vi "partsTracking_Create.vi"(6 "error in (no error)":errorcluster, 7 "dim":i32, 8 "index":i32, 9 "reference in":refnum<class "partsTracking.lvclass">) -> (0 "error out":errorcluster, 3 "reference out":refnum<class "partsTracking.lvclass">)   [LabVIEW 2016, in "partsTracking.lvclass"]
doc: "Constructor."
uses:
  partsTracking.lvclass
  C:/Program Files (x86)/National Instruments/LabVIEW 2016/vi.lib/addons/_AddQ/G#Object/G#Object.lvclass
  <vilib>/addons/_AddQ/G#Object/utils/G#Object_CreateMethod.ctl
  <vilib>/addons/_AddQ/G#Object/G#Object.lvclass
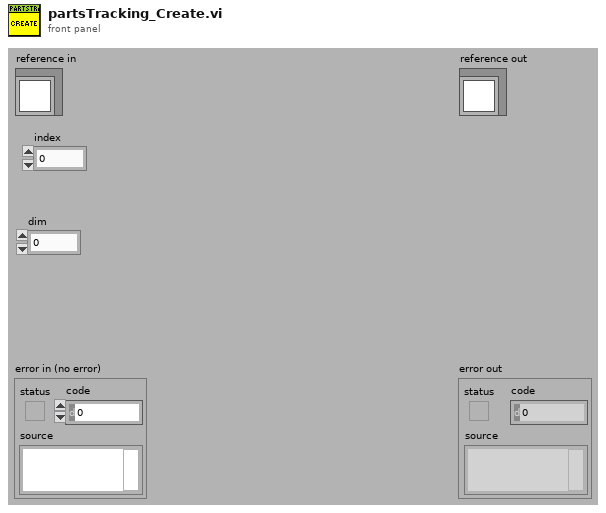
[diagram p1: front panel]
types:
  T1 = typedef "G#Object.lvclass/G#Object_CreateMethod.ctl" = enum16{"Create", "Create or look up existing", "Look up existing"}
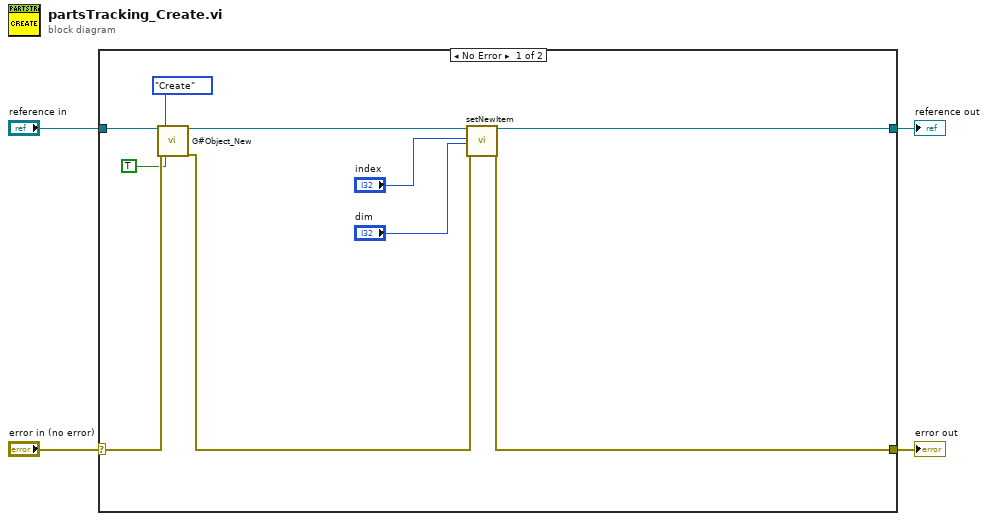
[diagram p0: block diagram]
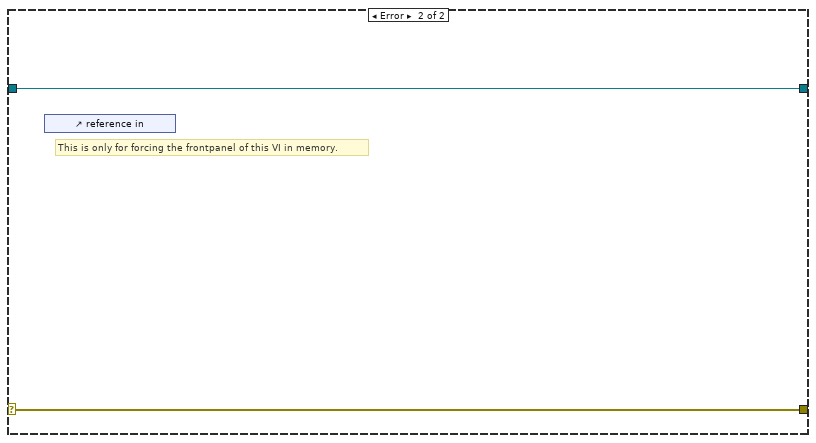
[diagram p2: hidden frame]
diagram:
  n1 = case shown="No Error" "error in (no error)" {
    selector: "error in (no error)" -> [w13 w16]
    tunnel: [w7 w16] -> w3
    tunnel: [w9 w15] -> w1
    tunnel: "reference in" -> [w14 w15]
    frame No Error {
      n2 = call <vilib>:"G#Object_New.vi"("reference in"=w14, "error in (no error)"=w13, "create method"=G#Object_CreateMethod."Create", "user counter (T)?"=TRUE ("User Counter")) -> ("reference out"=w10:refnum<class "partsTracking.lvclass">, "error out"=w8:errorcluster)  [unwired: 13 in, 1 out]
      n3 = call "setNewItem.vi"("reference in"=w10, "index"="index", "dim"="dim", "error in (no error)"=w8) -> ("reference out"=w9:refnum<class "partsTracking.lvclass">, "error out"=w7:errorcluster)  [unwired: 14 in]
    }
    frame Error {
      # "This is only for forcing the frontpanel of this VI in memory."
      n4 = control-ref of="reference in"() -> ()  [unwired: 1 out]
    }
  }
  "error out" <- w3
  "reference out" <- w1
